vi "test_stackHorizontally.vi"(11 "Test Case In":refnum<class "StackTests.lvclass">) -> (0 "error out":errorcluster, 3 "Test Case Out":refnum<class "StackTests.lvclass">)   [LabVIEW 2023, in "StackTests.lvclass"]
uses:
  StackTests.lvclass
  StackTests.lvclass/StackTests.ctl
  source/TLC_Geometry.lvlib
  <vilib>/Astemes/LUnit/Test Case.lvclass
  C:/Program Files (x86)/National Instruments/LabVIEW 2023/vi.lib/Astemes/LUnit/Test Case.lvclass
panel:
  in  "Numeric":dbl
  in  "btn":bool
  in  "firstItem":string
  in  "String":string
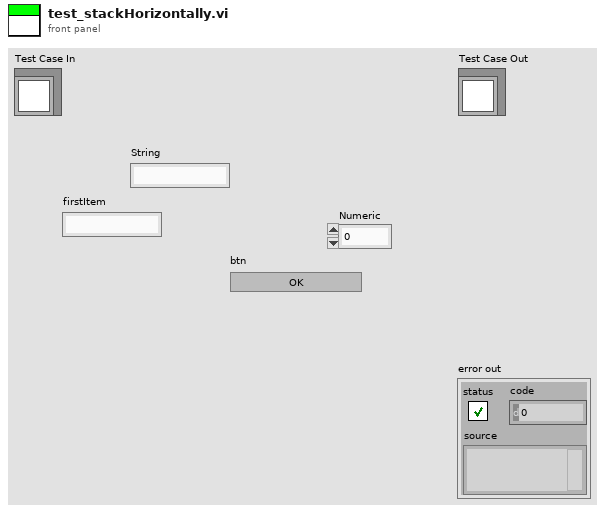
[diagram p1: front panel]
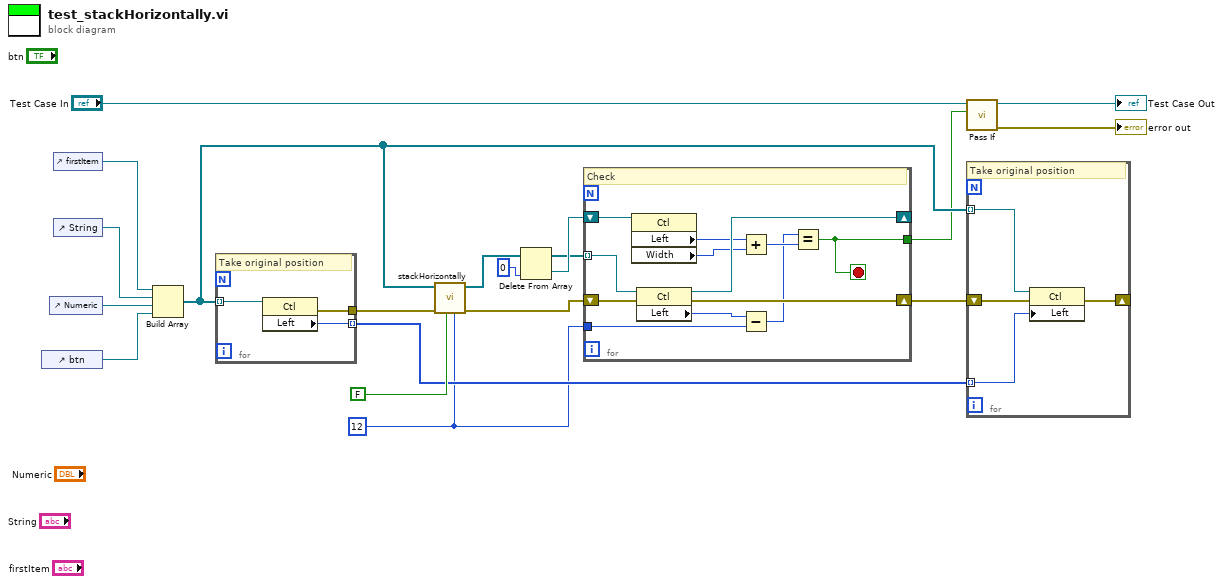
[diagram p0: block diagram]
diagram:
  w3 = u16 12 ("spacing")
  n1 = control-ref of="btn"() -> (w1:refnum<vi>)
  n2 = control-ref of="Numeric"() -> (w2:refnum<vi>)
  n3 = control-ref of="firstItem"() -> (w16:refnum<vi>)
  n4 = control-ref of="String"() -> (w15:refnum<vi>)
  n5 = Build Array(w16, w15, w2, w1) -> (w6:refnum<vi>[])
  n6 = for {
    tunnel: w6 -> [w22] mode=indexing
    tunnel: [w21] -> w4 mode=indexing
    tunnel: [w20] -> w14
    # "Take original position"
    n7 = property class="Ctl"(reference=w22) -> (error out=w20:errorcluster, "Left"=w21:i32)  [unwired: 1 in, 1 out]
  }
  n8 = call "stackHorizontally.vi"("spacing"=w3, "useControlBodyOnly"=FALSE, "error in (no error)"=w14, "refs"=w6) -> ("error out"=w12:errorcluster, "refs(dup)"=w9:refnum<vi>[])  [unwired: 6 in]
  n9 = Delete From Array(array=w9, index=0) -> (deleted portion=w10:refnum<vi>, array with subset deleted=w8:refnum<vi>[])  [unwired: 1 in]
  n10 = for {
    tunnel: w8 -> [w34] mode=indexing
    shift-right: [w32] -> w7
    shift-left: w12 -> [w33]
    shift-right: [w30] -> _
    shift-left: w10 -> [w31]
    tunnel: [w26] -> w5
    tunnel: w3 -> [w23]
    stop <- w26 stop-if-true
    # "Check"
    n11 = property class="Ctl"(reference=w31) -> ("Left"=w29:i32, "Width"=w28:u32)  [unwired: 1 in, 2 out]
    n12 = property class="Ctl"(reference=w34, error in=w33) -> (reference out=w30:refnum<vi>, error out=w32:errorcluster, "Left"=w25:i32)
    n13 = Add(x=w29, y=w28) -> (x+y=w27:u32)
    n14 = Subtract(x=w25, y=w23) -> (x-y=w24:i32)
    n15 = Equal?(x=w24, y=w27) -> (x = y?=w26:bool)
  }
  n16 = call <vilib>:"Pass If.vi"("Pass?"=w5, "LUnit Test Case In"="Test Case In") -> ("error out"=→"error out":errorcluster, "LUnit Test Case Out"=→"Test Case Out":refnum<class "StackTests.lvclass">)  [unwired: 8 in]
  n17 = for {
    tunnel: w6 -> [w38] mode=indexing
    tunnel: w4 -> [w37] mode=indexing
    shift-right: [w36] -> _
    shift-left: w7 -> [w35]
    # "Take original position"
    n18 = property class="Ctl"(reference=w38, error in=w35, "Left"=w37) -> (error out=w36:errorcluster)  [unwired: 1 out]
  }
